vi "Read PluginIniFilePath.vi"(8 "error in (no error)":errorcluster, 11 "BasePlugin in":refnum<class "BasePlugin.lvclass">) -> (0 "error out":errorcluster, 2 "PluginIniFilePath":path, 3 "BasePlugin out":refnum<class "BasePlugin.lvclass">)   [LabVIEW 2014, in "BaseClasses.lvlib" / "BasePlugin.lvclass"]
uses:
  BasePlugin.lvclass
  BasePlugin.lvclass/BasePlugin.ctl
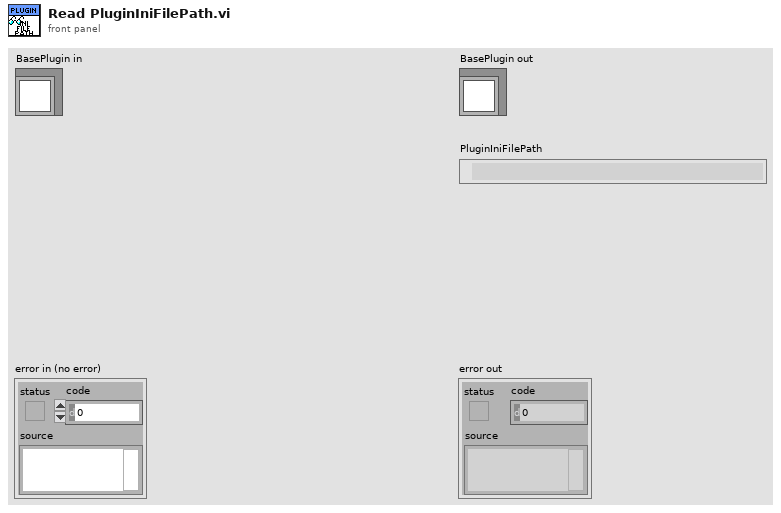
[diagram p1: front panel]
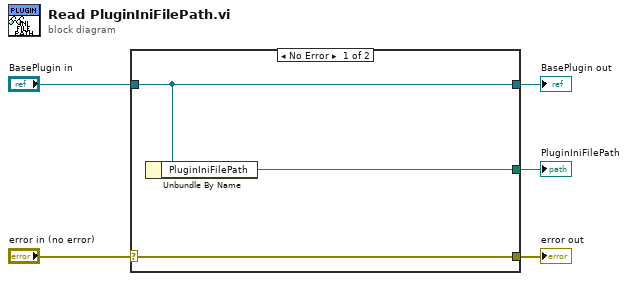
[diagram p0: block diagram]
diagram:
  n1 = case shown="No Error" "error in (no error)" {
    selector: "error in (no error)" -> [w8 w9]
    tunnel: [w8 w9] -> w4
    tunnel: [w7 w10] -> w2
    tunnel: "BasePlugin in" -> [w7 w10]
    tunnel: [w6 _] -> w1
    frame No Error {
      n2 = Unbundle By Name(w7) -> ("PluginIniFilePath"=w6:path)
    }
    frame Error {
    }
  }
  "error out" <- w4
  "BasePlugin out" <- w2
  "PluginIniFilePath" <- w1
